vi "Stop Server.vi"(8 "error in (no error)":errorcluster, 11 "OOP Server in":refnum<class "OOP Server.lvclass">) -> (0 "error out":errorcluster, 3 "OOP Server out":refnum<class "OOP Server.lvclass">)   [LabVIEW 2019, in "OOP Server.lvclass"]
uses:
  OOP Server.lvclass
  OOP Server.lvclass/OOP Server.ctl
  gRPC interface/gprc-lvsupport.lvlib
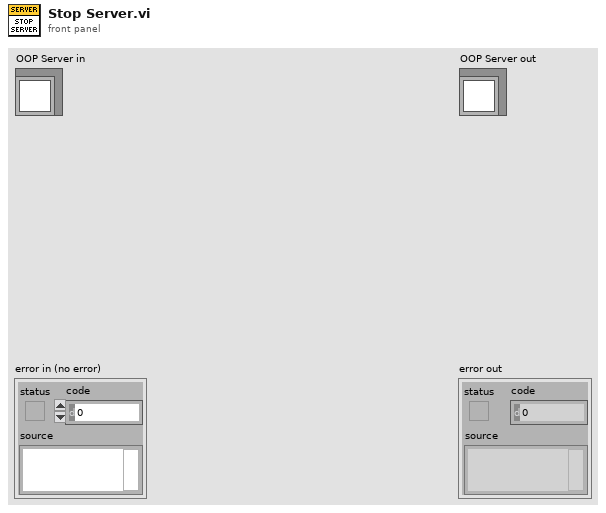
[diagram p1: front panel]
types:
  T1 = typedef "gprc-lvsupport.lvlib/grpcId.ctl" = u64
  T2 = typedef "OOP Server.lvclass/Server gRPC UEs.ctl" = cluster{"Invoke gRPC UEs":T3, "Query gRPC UEs":T3, "Register gRPC UEs":T3}
  T3 = typedef "gprc-lvsupport.lvlib/gRPCId Cluster UE.ctl" = refnum<user-event>
  T4 = typedef "OOP Server.lvclass/Server Internal UEs.ctl" = cluster{"Invoke Internal UE":refnum<user-event>, "Query Internal UE":refnum<user-event>, "Register Internal UE":refnum<user-event>}
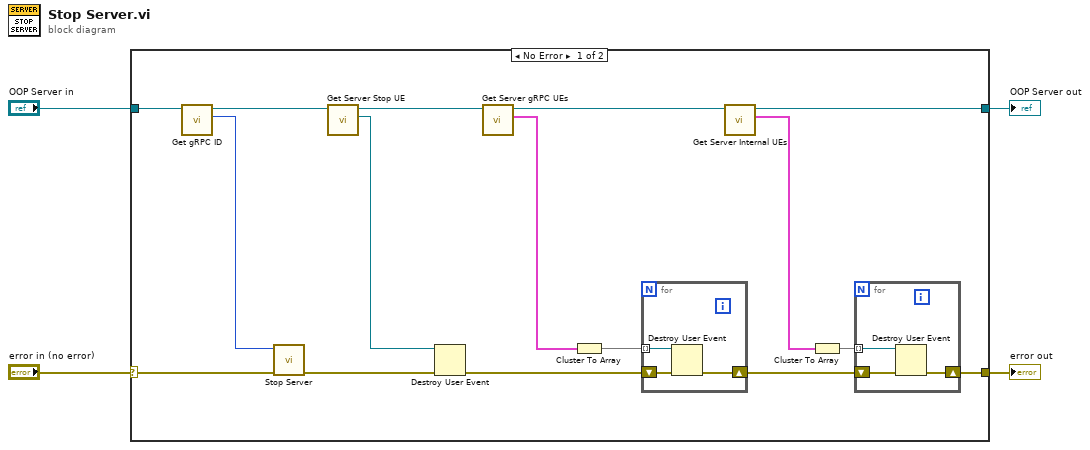
[diagram p0: block diagram]
diagram:
  n1 = case shown="No Error" "error in (no error)" {
    selector: "error in (no error)" -> [w19 w28]
    tunnel: [w5 w28] -> w3
    tunnel: [w12 w27] -> w1
    tunnel: "OOP Server in" -> [w20 w27]
    frame No Error {
      n2 = call "Get gRPC ID.vi"("OOP Server in"=w20) -> ("gRPC ID"=w18:T1, "OOP Server out"=w17:refnum<class "OOP Server.lvclass">)  [unwired: 9 in]
      n3 = call "Stop Server.vi"("error in (no error)"=w19, "Server Id"=w18) -> ("error out"=w16:errorcluster)  [unwired: 9 in]
      n4 = call "Get Server Stop UE.vi"("OOP Server in"=w17) -> ("Server Stop UE"=w15:refnum<user-event>, "OOP Server out"=w14:refnum<class "OOP Server.lvclass">)  [unwired: 9 in]
      n5 = Destroy User Event(user event=w15, error in=w16) -> (error out=w9:errorcluster)
      n6 = call "Get Server gRPC UEs.vi"("OOP Server in"=w14) -> ("Server gRPC UEs"=w11:T2, "OOP Server out"=w13:refnum<class "OOP Server.lvclass">)  [unwired: 9 in]
      n7 = Cluster To Array(cluster=w11) -> (array=w10:T3[])
      n8 = for {
        tunnel: w10 -> [w26] mode=indexing
        shift-right: [w24] -> w8
        shift-left: w9 -> [w25]
        n9 = Destroy User Event(user event=w26, error in=w25) -> (error out=w24:errorcluster)
      }
      n10 = call "Get Server Internal UEs.vi"("OOP Server in"=w13) -> ("Server Internal UEs"=w7:T4, "OOP Server out"=w12:refnum<class "OOP Server.lvclass">)  [unwired: 9 in]
      n11 = Cluster To Array(cluster=w7) -> (array=w6:refnum<user-event>[])
      n12 = for {
        tunnel: w6 -> [w23] mode=indexing
        shift-right: [w21] -> w5
        shift-left: w8 -> [w22]
        n13 = Destroy User Event(user event=w23, error in=w22) -> (error out=w21:errorcluster)
      }
    }
    frame Error {
    }
  }
  "error out" <- w3
  "OOP Server out" <- w1
